vi "Decode HydroHarp v2 TTT Data.vi"(8 "oflcorr_in":u64, 11 "rawbits":u32) -> (0 "oflcorr_out":u64, 1 "channel":u8, 2 "dtime":u32, 3 "truetime":u64, 4 "markercode":u32)   [LabVIEW 2021, in "PTU Files.lvlib"]
uses:
  PTU Files.lvlib
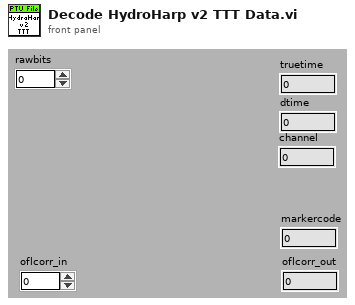
[diagram p1: front panel]
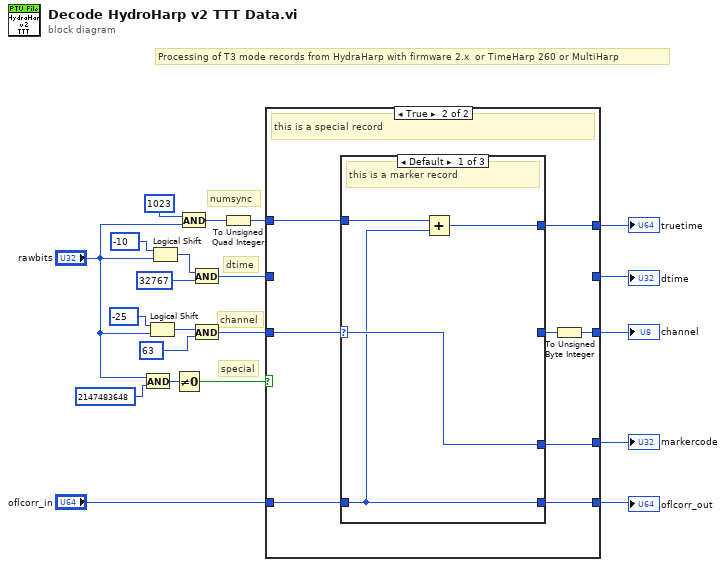
[diagram p0: block diagram]
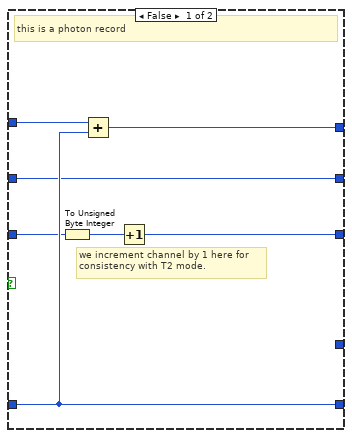
[diagram p2: hidden frame]
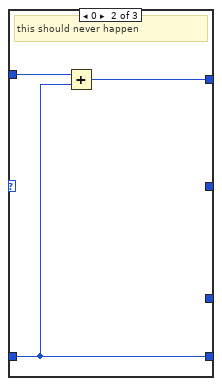
[diagram p3: hidden frame]
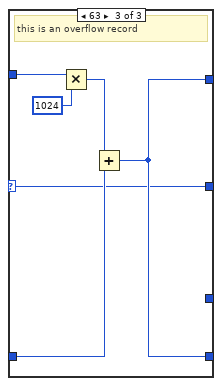
[diagram p4: hidden frame]
diagram:
  # "special"
  # "Processing of T3 mode records from HydraHarp with firmware 2.x  or TimeHarp 260 or MultiHarp"
  # "dtime"
  # "channel"
  # "numsync"
  n1 = And(x="rawbits", y=u32 2147483648 ("x")) -> (x .and. y?=w7:u32)
  n2 = Logical Shift(y=-25, x="rawbits") -> (x << y=w15:u32)
  n3 = Logical Shift(y=-10, x="rawbits") -> (x << y=w18:u32)
  n4 = Not Equal To 0?(x=w7) -> (x != 0?=w4:bool)
  n5 = And(x=u32 1023, y="rawbits") -> (x .and. y?=w2:u32)
  n6 = And(x=w18, y=u32 32767 ("x")) -> (x .and. y?=w16:u32)
  n7 = And(x=w15, y=u32 63 ("x")) -> (x .and. y?=w3:u32)
  n8 = To Unsigned Quad Integer(1:w2) -> (0:w1:u64)
  n9 = case shown="True" w4 {
    tunnel: w1 -> [w25 w31]
    tunnel: "oflcorr_in" -> [w28 w36]
    tunnel: [w28 w35] -> w12
    tunnel: [_ w34] -> w11
    tunnel: w16 -> [w26 _]
    tunnel: [w27 w32] -> w9
    tunnel: [w26 _] -> w8
    tunnel: [w23 w29] -> w10
    tunnel: w3 -> [w24 w33]
    frame False {
      # "we increment channel by 1 here for\nconsistency with T2 mode."
      # "this is a photon record"
      n10 = To Unsigned Byte Integer(number=w24) -> (unsigned 8bit integer=w22:u8)
      n11 = Add(x=w25, y=w28) -> (x+y=w27:u64)
      n12 = Increment(x=w22) -> (x+1=w23:u8)
    }
    frame True {
      # "this is a special record"
      n13 = case shown="Default" w33 {
        selector: w33 -> [w40 _ w44]
        tunnel: w36 -> [w38 w42 w46]
        tunnel: [w38 w42 w45] -> w35
        tunnel: [w40 _ _] -> w34
        tunnel: [w37 w41 w45] -> w32
        tunnel: w31 -> [w39 w43 w49]
        tunnel: [_ _ w44] -> w30
        frame Default {
          # "this is a marker record"
          n14 = Add(x=w39, y=w38) -> (x+y=w37:u64)
        }
        frame 0 {
          # "this should never happen"
          n15 = Add(x=w43, y=w42) -> (x+y=w41:u64)
        }
        frame 63 {
          # "this is an overflow record"
          n16 = Multiply(x=w49, y=u64 1024 ("x")) -> (x*y=w47:u64)
          n17 = Add(x=w47, y=w46) -> (x+y=w45:u64)
        }
      }
      n18 = To Unsigned Byte Integer(number=w30) -> (unsigned 8bit integer=w29:u8)
    }
  }
  "channel" <- w10
  "truetime" <- w9
  "markercode" <- w11
  "oflcorr_out" <- w12
  "dtime" <- w8
